vi "Read Core OOB RX.vi"(8 "error in (no error)":errorcluster, 11 "CIFCorePlugin in":refnum<class "CIFCorePlugin.lvclass">) -> (0 "error out":errorcluster, 3 "CIFCorePlugin out":refnum<class "CIFCorePlugin.lvclass">)   [LabVIEW 2021, in "CIFCorePlugin.lvclass"]
uses:
  CIFCorePlugin.lvclass
  CIFCorePlugin.lvclass/CIFCorePlugin.ctl
  <vilib>/CIF Foundation/CIF Out of Band Commands/CIFOutOfBand.lvclass/CIFOutOfBand.ctl
  Typedef/Energized States.ctl
  OOB/OOB_Rx/CIFCoreOOB_Rx.lvclass/CIFCoreOOB_Rx.ctl
  Channels/CIFChannelMng/CIFChannelMng.lvclass/CIFChannelMng.ctl
  <vilib>/CIF Foundation/CIF Channels Core/CIFChannels/CIFChannels.lvclass/CIFChannels.ctl
  OOB/OOB_Rx/Private/Read Payload.vi
  Channels/CIFChannelMng/Utilities/Get Channel Index by Name.vi
  <vilib>/CIF Foundation/CIF Channels Core/CIFChannels/Accessors/Read Channel State.vi
  Channels/CIFChannelMng/OOB/OOB_Tx/Send/Update Channel List Command.vi
  <vilib>/CIF Foundation/CIF Out of Band Commands/Commit Commands.vi
  <vilib>/CIF Foundation/CIF Channels Core/CIFChannels/Accessors/Read Tag Forced.vi
  Channels/CIFChannelMng/SubVIs/Add Error Channel Manager.vi
  Channels/CIFChannelMng/OOB/OOB_Tx/Send/FIFO Publisher Return Command.vi
  Channels/CIFChannelMng/SubVIs/Get Original FIFO Channel Name.vi
  <vilib>/CIF Foundation/CIF Out of Band Commands/Read Commands.vi
  OOB/OOB_Rx/Private/Command Settings.vi
  <vilib>/CIF Foundation/CIF Out of Band Commands/Accessors/Read Local OOB Data.vi
  <vilib>/CIF Foundation/CIF Channels Core/ChannelCommon/Utilities/Add Error.vi
  <vilib>/CIF Foundation/CIF Out of Band Commands/Queue Command.vi
  <vilib>/CIF Foundation/CIF Out of Band Commands/Utilities/Command to Bitwise Command.vi
  <vilib>/CIF Foundation/CIF Utilities/Errors/Append Error Location.vi
  OOB/OOB_Rx/CIFCoreOOB_Rx.lvclass
  C:/Program Files/National Instruments/LabVIEW 2021/vi.lib/CIF Foundation/CIF Out of Band Commands/CIFOutOfBand.lvclass
  Channels/CIFChannelMng/OOB/OOB_Tx/ChnMngOOB_Tx.lvclass
  <vilib>/CIF Foundation/CIF Channels Core/CIFChannels/Core/Set Force.vi
  <vilib>/CIF Foundation/CIF Channels Core/CIFChannels/CIFChannels.lvclass
  Channels/CIFChannelMng/CIFChannelMng.lvclass
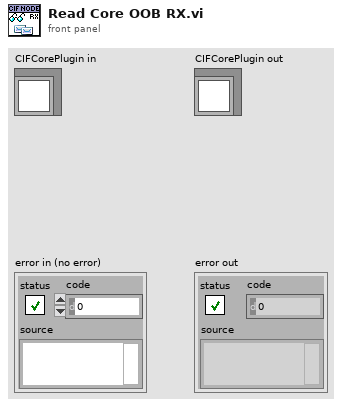
[diagram p1: front panel]
types:
  T1 = typedef "CIFCorePlugin.lvclass/Energized States.ctl" = enum16{"Listen", "Prepare", "Execute", "Housekeep", "Cleanup", "Destroy"}
  T2 = typedef "CIFCoreOOB_Rx.lvclass/OOB Core Commands.ctl" = enum8{"Start", "Pause", "Stop", "RefreshStats", "UpdateConfig", "Update Clock Map", "Connect Channel", "Force Channel", "Add Publisher Instance", "Remove Publisher Instance"}
  T3 = typedef "Time_CIF_U.lvlib/Clock Conversion Map.ctl" = map{u8, cluster{"Last Reset":i64, "Offset Pair":T4, "Slope":dbl, "1/Slope":dbl}}
  T4 = typedef "Time_CIF_U.lvlib/Timestamp Pair.ctl" = cluster{"System Time":i64, "External Time":i64}
  T5 = typedef "CIFCoreOOB_Rx.lvclass/Channel Connection Data.ctl" = cluster{"Publisher Name":string, "Subscriber Name":string, "Connection Data":u8[]}
  T6 = typedef "CIFCoreOOB_Rx.lvclass/Channel Fault Data.ctl" = cluster{"Channel Name":string, "Force Data":u8[], "Force Active":bool}
  T7 = typedef "CIFCoreOOB_Rx.lvclass/FIFO Publisher.ctl" = cluster{"Publisher Name":string, "New FIFO Instance Config":T8}
  T8 = typedef "ChannelCommon.lvlib/New FIFO Instance Configuration.ctl" = cluster{"Primary":bool, "Backpressure":bool, "Message/FIFO Override":u32}
  T9 = typedef "ChnMngOOB_Tx.lvclass/FIFO Publisher Return.ctl" = cluster{"FIFO Pub Name":string, "error":errorcluster, "Added":bool}
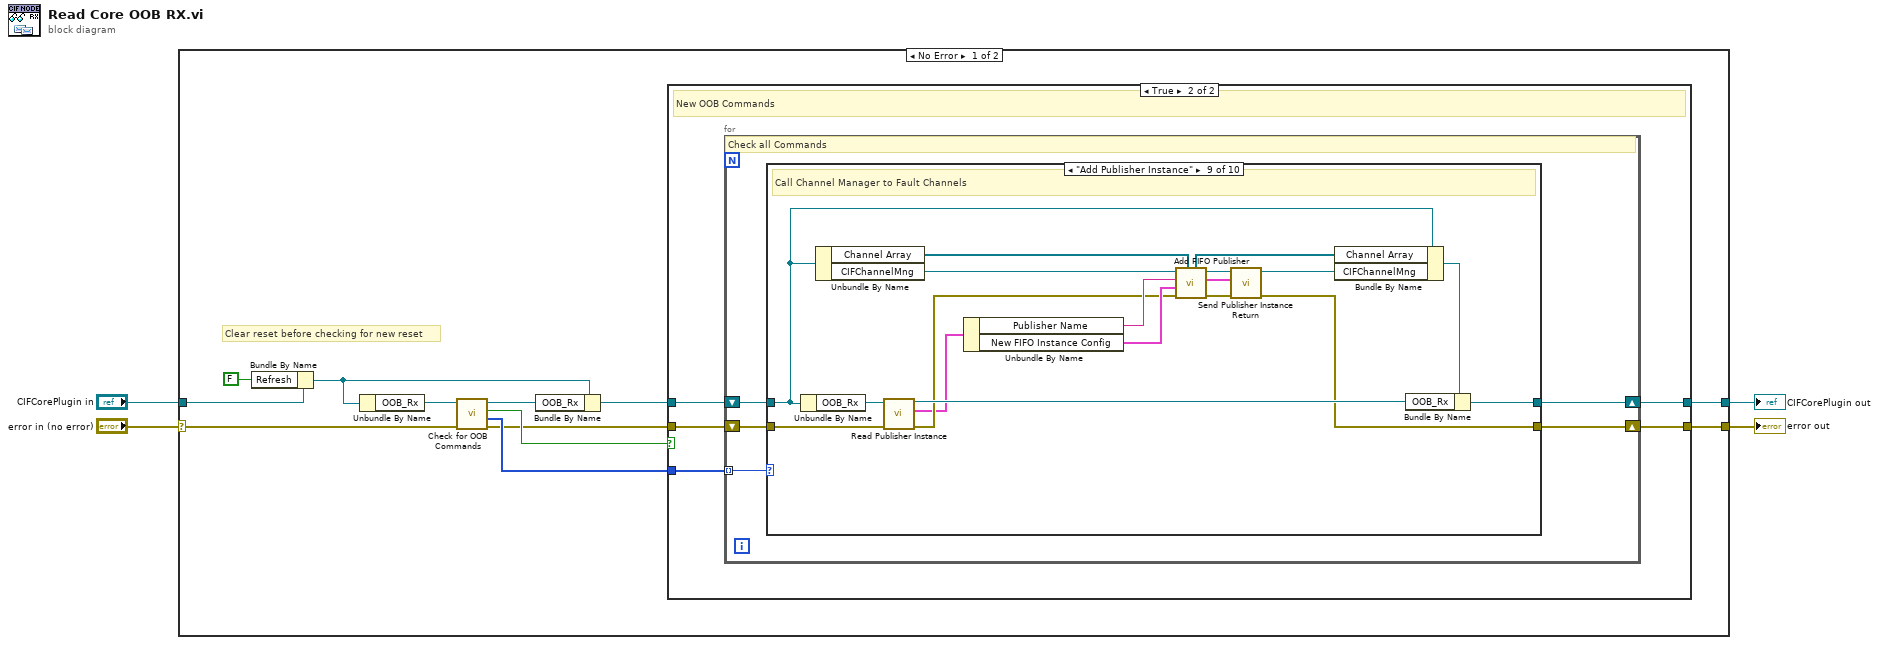
[diagram p0: block diagram]
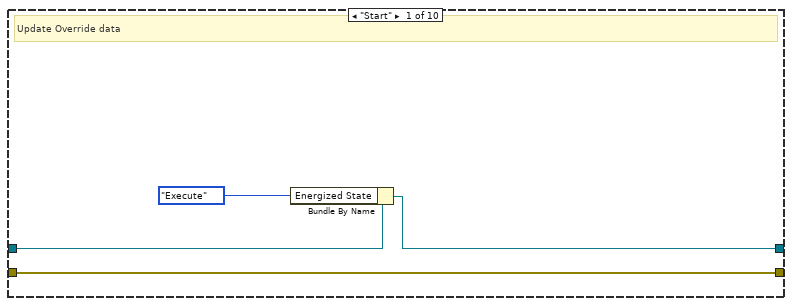
[diagram p3: hidden frame]
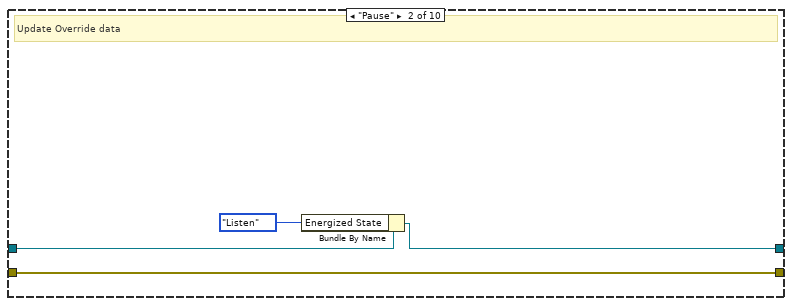
[diagram p4: hidden frame]
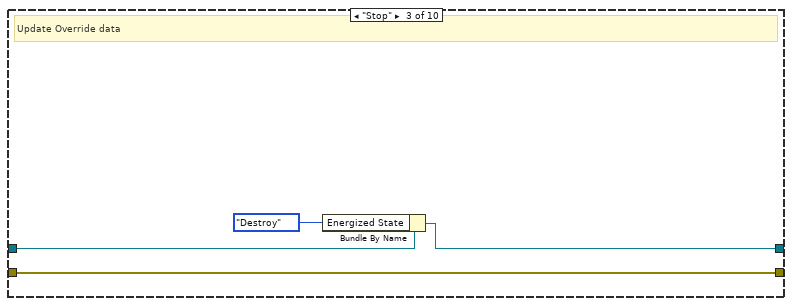
[diagram p5: hidden frame]
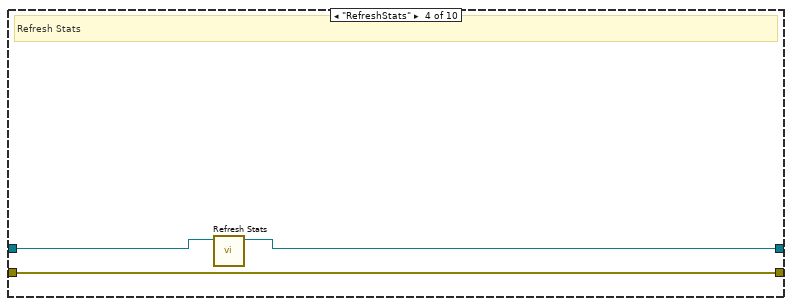
[diagram p6: hidden frame]
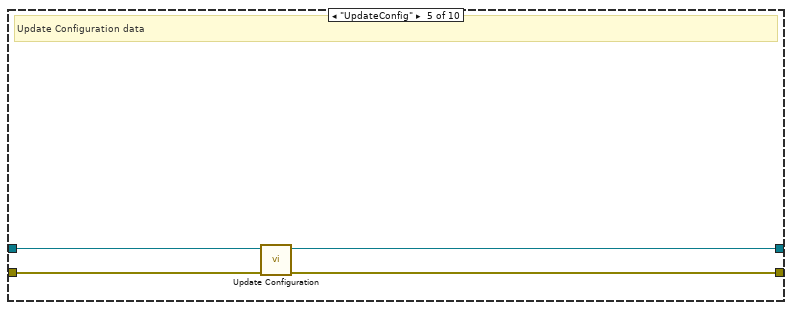
[diagram p7: hidden frame]
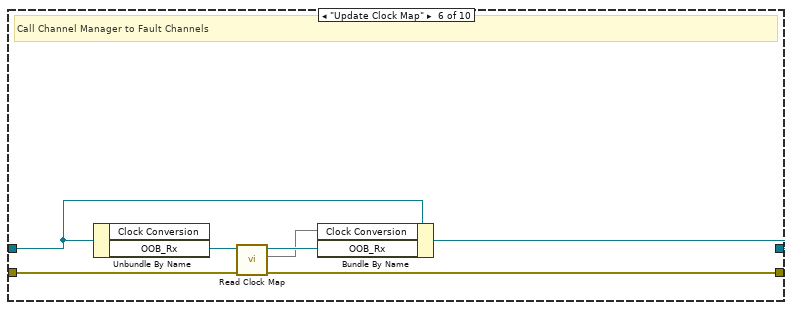
[diagram p8: hidden frame]
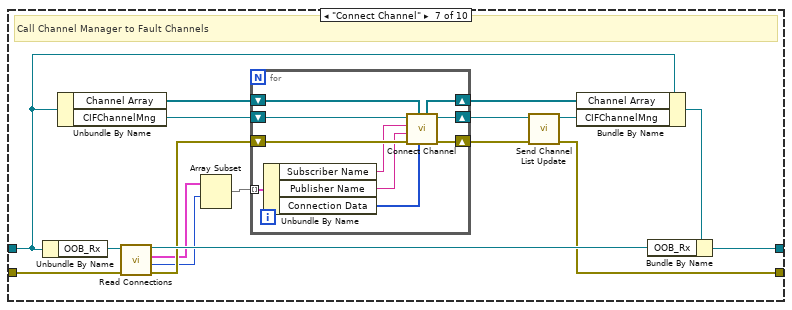
[diagram p9: hidden frame]
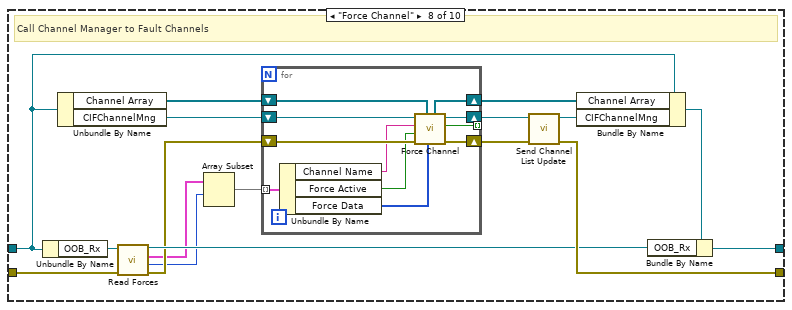
[diagram p10: hidden frame]
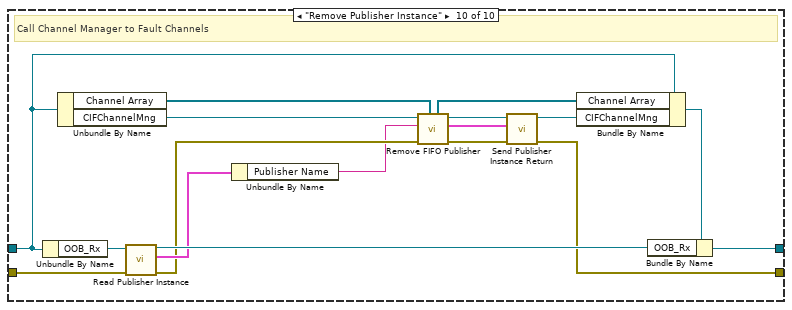
[diagram p11: hidden frame]
diagram:
  n1 = case shown="No Error" "error in (no error)" {
    selector: "error in (no error)" -> [w16 w146]
    tunnel: [w7 w146] -> w1
    tunnel: [w8 w145] -> w2
    tunnel: "CIFCorePlugin in" -> [w11 w145]
    frame No Error {
      # "Clear reset before checking for new reset"
      n2 = Bundle By Name(cluster=w11, "Refresh"=FALSE ("Running Internal Data.Refresh")) -> (w10:refnum<class "CIFCorePlugin.lvclass">)
      n3 = Unbundle By Name(w10) -> ("OOB_Rx"=w6:refnum<class "CIFCoreOOB_Rx.lvclass">)
      n4 = call "Check for OOB Commands.vi"("error in (no error)"=w16, "CoreOOB_Rx in"=w6) -> ("error out"=w13:errorcluster, "Commands"=w14:T2[], "New Commands"=w15:bool, "CoreOOB_Rx out"=w5:refnum<class "CIFCoreOOB_Rx.lvclass">)  [unwired: 6 in]
      n5 = Bundle By Name(cluster=w10, "OOB_Rx"=w5) -> (w9:refnum<class "CIFCorePlugin.lvclass">)
      n6 = case shown="True" w15 {
        tunnel: w14 -> [_ w23]
        tunnel: w9 -> [w18 w22]
        tunnel: [w18 w20] -> w8
        tunnel: w13 -> [w17 w21]
        tunnel: [w17 w19] -> w7
        frame False {
          # "No new OOB Commands"
        }
        frame True {
          # "New OOB Commands"
          n7 = for {
            tunnel: w23 -> [w28] mode=indexing
            shift-right: [w25] -> w20
            shift-left: w22 -> [w26]
            shift-right: [w24] -> w19
            shift-left: w21 -> [w27]
            # "Check all Commands"
            n8 = case shown="\"Add Publisher Instance\"" w28 {
              tunnel: w27 -> [w29 w36 w40 w41 w46 w53 w68 w92 w120 w140]
              tunnel: w26 -> [w30 w35 w39 w43 w47 w54 w63 w96 w126 w143]
              tunnel: [w32 w34 w38 w42 w45 w52 w71 w98 w127 w144] -> w25
              tunnel: [w29 w36 w40 w41 w44 w51 w60 w94 w110 w136] -> w24
              frame "Start" {
                # "Update Override data"
                n9 = Bundle By Name(cluster=w30, "Energized State"=Energized_States."Execute" ("Energized States in")) -> (w32:refnum<class "CIFCorePlugin.lvclass">)
              }
              frame "Pause" {
                # "Update Override data"
                n10 = Bundle By Name(cluster=w35, "Energized State"=Energized_States."Listen" ("Energized States in")) -> (w34:refnum<class "CIFCorePlugin.lvclass">)
              }
              frame "Stop" {
                # "Update Override data"
                n11 = Bundle By Name(cluster=w39, "Energized State"=Energized_States."Destroy" ("Energized States in")) -> (w38:refnum<class "CIFCorePlugin.lvclass">)
              }
              frame "RefreshStats" {
                # "Refresh Stats"
                n12 = call "Refresh Stats.vi"("CIFCorePlugin in"=w43) -> ("CIFCorePlugin out"=w42:refnum<class "CIFCorePlugin.lvclass">)  [unwired: 10 in]
              }
              frame "UpdateConfig" {
                # "Update Configuration data"
                n13 = call-dynamic "Update Configuration.vi"("error in (no error)"=w46, "CIFTemplateNode in"=w47) -> ("error out"=w44:errorcluster, "CIFTemplateNode out"=w45:refnum<class "CIFCorePlugin.lvclass">)  [unwired: 8 in]
              }
              frame "Update Clock Map" {
                # "Call Channel Manager to Fault Channels"
                n14 = Unbundle By Name(w54) -> ("OOB_Rx"=w50:refnum<class "CIFCoreOOB_Rx.lvclass">)  [unwired: 1 out]
                n15 = call "Read Clock Map.vi"("error in"=w53, "CoreOOB_Rx in"=w50) -> ("error out"=w51:errorcluster, "Clock Conversion"=w48:T3, "CoreOOB_Rx out"=w49:refnum<class "CIFCoreOOB_Rx.lvclass">)  [unwired: 7 in]
                n16 = Bundle By Name(cluster=w54, "Clock Conversion"=w48, "OOB_Rx"=w49) -> (w52:refnum<class "CIFCorePlugin.lvclass">)
              }
              frame "Connect Channel" {
                # "Call Channel Manager to Fault Channels"
                n17 = Unbundle By Name(w63) -> ("OOB_Rx"=w69:refnum<class "CIFCoreOOB_Rx.lvclass">)
                n18 = Unbundle By Name(w63) -> ("Channel Array"=w56:refnum<class "CIFChannels.lvclass">[], "CIFChannelMng"=w70:refnum<class "CIFChannelMng.lvclass">)
                n19 = call "Read Connections.vi"("error in"=w68, "CoreOOB_Rx in"=w69) -> ("error out"=w61:errorcluster, "Offset"=w57:i32, "Connections"=w59:T5[], "CoreOOB_Rx out"=w67:refnum<class "CIFCoreOOB_Rx.lvclass">)  [unwired: 6 in]
                n20 = Array Subset(array=w59, index=w57) -> (w58:T5[])  [unwired: 1 in]
                n21 = for {
                  tunnel: w58 -> [w81] mode=indexing
                  shift-right: [w79] -> w66
                  shift-left: w70 -> [w80]
                  shift-right: [w78] -> w65
                  shift-left: w61 -> [w77]
                  shift-right: [w72] -> w55
                  shift-left: w56 -> [w73]
                  n22 = Unbundle By Name(w81) -> ("Subscriber Name"=w76:string, "Publisher Name"=w75:string, "Connection Data"=w74:u8[])
                  n23 = call "Connect Channel.vi"("Custom Channel Config Data"=w74, "Channel Array in"=w73, "error in (no error)"=w77, "Publisher Name"=w75, "Subscriber Name"=w76, "CIFChannelMng in"=w80) -> ("error out"=w78:errorcluster, "CIFChannelMng out"=w79:refnum<class "CIFChannelMng.lvclass">, "Channel Array out"=w72:refnum<class "CIFChannels.lvclass">[])  [unwired: 2 in, 1 out]
                }
                n24 = call "Send Channel List Update.vi"("error in (no error)"=w65, "CIFChannelMng in"=w66) -> ("error out"=w60:errorcluster, "CIFChannelMng out"=w64:refnum<class "CIFChannelMng.lvclass">)  [unwired: 8 in]
                n25 = Bundle By Name(cluster=w63, "Channel Array"=w55, "CIFChannelMng"=w64) -> (w62:refnum<class "CIFCorePlugin.lvclass">)
                n26 = Bundle By Name(cluster=w62, "OOB_Rx"=w67) -> (w71:refnum<class "CIFCorePlugin.lvclass">)
              }
              frame "Force Channel" {
                # "Call Channel Manager to Fault Channels"
                n27 = Unbundle By Name(w96) -> ("OOB_Rx"=w93:refnum<class "CIFCoreOOB_Rx.lvclass">)
                n28 = Unbundle By Name(w96) -> ("Channel Array"=w83:refnum<class "CIFChannels.lvclass">[], "CIFChannelMng"=w90:refnum<class "CIFChannelMng.lvclass">)
                n29 = call "Read Forces.vi"("error in"=w92, "CoreOOB_Rx in"=w93) -> ("error out"=w89:errorcluster, "Offset"=w84:i32, "Forces"=w86:T6[], "CoreOOB_Rx out"=w91:refnum<class "CIFCoreOOB_Rx.lvclass">)  [unwired: 6 in]
                n30 = Array Subset(array=w86, index=w84) -> (w85:T6[])  [unwired: 1 in]
                n31 = for {
                  tunnel: w85 -> [w107] mode=indexing
                  shift-right: [w103] -> w87
                  shift-left: w90 -> [w109]
                  shift-right: [w102] -> w88
                  shift-left: w89 -> [w108]
                  tunnel: [w101] -> _ mode=indexing
                  shift-right: [w99] -> w82
                  shift-left: w83 -> [w100]
                  n32 = Unbundle By Name(w107) -> ("Channel Name"=w106:string, "Force Active"=w105:bool, "Force Data"=w104:u8[])
                  n33 = call "Force Channel.vi"("Force Data"=w104, "Channel Array in"=w100, "error in (no error)"=w108, "Force Active"=w105, "Channel Name"=w106, "CIFChannelMng in"=w109) -> ("error out"=w102:errorcluster, "Update OOB"=w101:bool, "CIFChannelMng out"=w103:refnum<class "CIFChannelMng.lvclass">, "Channel Array out"=w99:refnum<class "CIFChannels.lvclass">[])  [unwired: 2 in]
                }
                n34 = call "Send Channel List Update.vi"("error in (no error)"=w88, "CIFChannelMng in"=w87) -> ("error out"=w94:errorcluster, "CIFChannelMng out"=w97:refnum<class "CIFChannelMng.lvclass">)  [unwired: 8 in]
                n35 = Bundle By Name(cluster=w96, "Channel Array"=w82, "CIFChannelMng"=w97) -> (w95:refnum<class "CIFCorePlugin.lvclass">)
                n36 = Bundle By Name(cluster=w95, "OOB_Rx"=w91) -> (w98:refnum<class "CIFCorePlugin.lvclass">)
              }
              frame "Add Publisher Instance" {
                # "Call Channel Manager to Fault Channels"
                n37 = Unbundle By Name(w126) -> ("OOB_Rx"=w121:refnum<class "CIFCoreOOB_Rx.lvclass">)
                n38 = Unbundle By Name(w126) -> ("Channel Array"=w113:refnum<class "CIFChannels.lvclass">[], "CIFChannelMng"=w124:refnum<class "CIFChannelMng.lvclass">)
                n39 = call "Read Publisher Instance.vi"("error in"=w120, "CoreOOB_Rx in"=w121) -> ("error out"=w118:errorcluster, "Publisher Instance"=w117:T7, "CoreOOB_Rx out"=w119:refnum<class "CIFCoreOOB_Rx.lvclass">)  [unwired: 7 in]
                n40 = Unbundle By Name(w117) -> ("Publisher Name"=w123:string, "New FIFO Instance Config"=w122:T8)
                n41 = call "Add FIFO Publisher.vi"("Channel Array in"=w113, "error in (no error)"=w118, "New FIFO Instance Config"=w122, "Channel Name"=w123, "CIFChannelMng in"=w124) -> ("error out"=w115:errorcluster, "FIFO Publisher"=w114:T9, "CIFChannelMng out"=w116:refnum<class "CIFChannelMng.lvclass">, "Channel Array out"=w112:refnum<class "CIFChannels.lvclass">[])  [unwired: 2 in, 1 out]
                n42 = call "Send Publisher Instance Return.vi"("error in (no error)"=w115, "Publisher Instance"=w114, "CIFChannelMng in"=w116) -> ("error out"=w110:errorcluster, "CIFChannelMng out"=w111:refnum<class "CIFChannelMng.lvclass">)  [unwired: 7 in]
                n43 = Bundle By Name(cluster=w126, "Channel Array"=w112, "CIFChannelMng"=w111) -> (w125:refnum<class "CIFCorePlugin.lvclass">)
                n44 = Bundle By Name(cluster=w125, "OOB_Rx"=w119) -> (w127:refnum<class "CIFCorePlugin.lvclass">)
              }
              frame "Remove Publisher Instance" {
                # "Call Channel Manager to Fault Channels"
                n45 = Unbundle By Name(w143) -> ("OOB_Rx"=w141:refnum<class "CIFCoreOOB_Rx.lvclass">)
                n46 = Unbundle By Name(w143) -> ("Channel Array"=w129:refnum<class "CIFChannels.lvclass">[], "CIFChannelMng"=w135:refnum<class "CIFChannelMng.lvclass">)
                n47 = call "Read Publisher Instance.vi"("error in"=w140, "CoreOOB_Rx in"=w141) -> ("error out"=w134:errorcluster, "Publisher Instance"=w138:T7, "CoreOOB_Rx out"=w139:refnum<class "CIFCoreOOB_Rx.lvclass">)  [unwired: 7 in]
                n48 = Unbundle By Name(w138) -> ("Publisher Name"=w133:string)
                n49 = call "Remove FIFO Publisher.vi"("Channel Array in"=w129, "error in (no error)"=w134, "Channel Name"=w133, "CIFChannelMng in"=w135) -> ("error out"=w132:errorcluster, "FIFO Publisher"=w131:T9, "CIFChannelMng out"=w130:refnum<class "CIFChannelMng.lvclass">, "Channel Array out"=w128:refnum<class "CIFChannels.lvclass">[])  [unwired: 3 in, 1 out]
                n50 = call "Send Publisher Instance Return.vi"("error in (no error)"=w132, "Publisher Instance"=w131, "CIFChannelMng in"=w130) -> ("error out"=w136:errorcluster, "CIFChannelMng out"=w137:refnum<class "CIFChannelMng.lvclass">)  [unwired: 7 in]
                n51 = Bundle By Name(cluster=w143, "Channel Array"=w128, "CIFChannelMng"=w137) -> (w142:refnum<class "CIFCorePlugin.lvclass">)
                n52 = Bundle By Name(cluster=w142, "OOB_Rx"=w139) -> (w144:refnum<class "CIFCorePlugin.lvclass">)
              }
            }
          }
        }
      }
    }
    frame Error {
    }
  }
  "error out" <- w1
  "CIFCorePlugin out" <- w2
